vi "Get System Name.vi"() -> (3 "System Name":string)   [LabVIEW 2016]
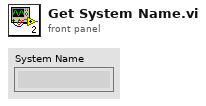
[diagram p1: front panel]
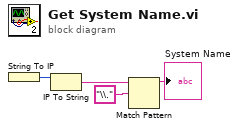
[diagram p0: block diagram]
diagram:
  n1 = String To IP() -> (0:w4:u32)  [unwired: 1 in]
  n2 = IP To String(2:w4) -> (0:w2:string)  [unwired: 1 in]
  n3 = Match Pattern(string=w2, regular expression="\\.") -> (before substring=→"System Name":string)  [unwired: 1 in, 3 out]
